vi "Actor Core.vi"(8 "error in":errorcluster, 11 "Device Manager in":refnum<class "Device Manager.lvclass">) -> (0 "error out":errorcluster, 3 "Actor out":refnum<class "Actor.lvclass">)   [LabVIEW 2020, in "Device Manager.lvlib" / "Device Manager.lvclass"]
doc: "<p>(<strong>Filename</strong>: <span class=\"dnl\">Actor Framework.lvlib:Actor.lvclass:Actor Core.vi</span>)</p>\n<p>Receives messages to the actor, reacts to them, and initiates any error handling that may shut the actor down.</p>\n<p>Descendant classes may override this VI to append parallel tasks for the actor to complete while it handles messages. Overrides use the <a href=\"nihelplauncher://docs/csh?context=lvcore_glang_udclass\">Call Parent Class Method</a> node.</p>"
uses:
  Device Manager.lvclass
  C:/Program Files/National Instruments/LabVIEW 2026/vi.lib/ActorFramework/Actor/Actor.lvclass
  <vilib>/ActorFramework/Actor/Actor.lvclass
  Front Panel Emulator/Front Panel Emulator.lvclass
  Servo Motor Emulator/Servo Motor Emulator.lvclass
  Device Manager.lvclass/Device Manager.ctl
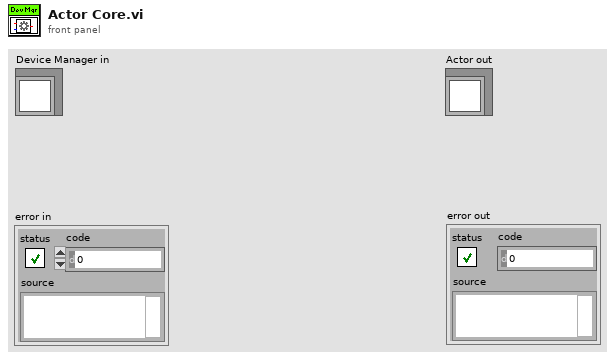
[diagram p1: front panel]
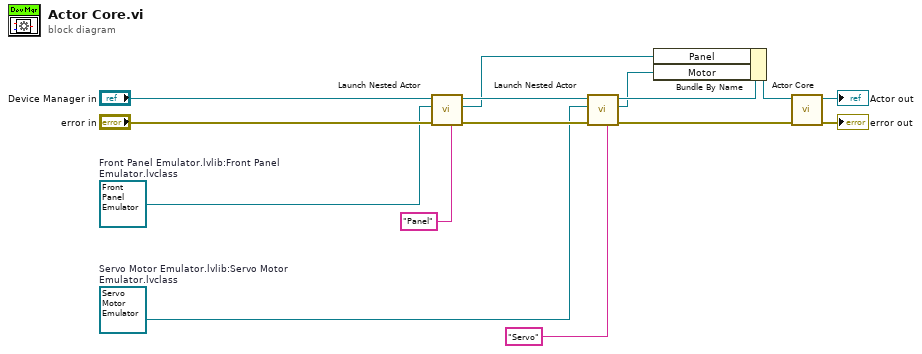
[diagram p0: block diagram]
diagram:
  w4 = refnum<class "Servo Motor Emulator.lvclass"> refnum  # Servo Motor Emulator.lvlib:Servo Motor Emulator.lvclass
  w5 = refnum<class "Front Panel Emulator.lvclass"> refnum  # Front Panel Emulator.lvlib:Front Panel Emulator.lvclass
  n1 = call <vilib>:"Launch Nested Actor.vi"("Debug Alias"="Panel", "error in (no error)"="error in", "Nested Actor"=w5, "Caller Actor in"="Device Manager in") -> ("error out"=w11:errorcluster, "Nested Actor's Enqueuer"=w6:refnum<class "Message Enqueuer.lvclass">, "Caller Actor out"=w10:refnum<class "Device Manager.lvclass">)  [unwired: 5 in]
  n2 = call <vilib>:"Launch Nested Actor.vi"("Debug Alias"="Servo", "error in (no error)"=w11, "Nested Actor"=w4, "Caller Actor in"=w10) -> ("error out"=w12:errorcluster, "Nested Actor's Enqueuer"=w7:refnum<class "Message Enqueuer.lvclass">, "Caller Actor out"=w9:refnum<class "Device Manager.lvclass">)  [unwired: 5 in]
  n3 = Bundle By Name(cluster=w9, "Panel"=w6, "Motor"=w7) -> (w8:refnum<class "Device Manager.lvclass">)
  n4 = call-parent "Actor Core.vi"("error in"=w12, "Actor in"=w8) -> ("error out"=→"error out":errorcluster, "Actor out"=→"Actor out":refnum<class "Actor.lvclass">)  [unwired: 8 in]
